vi "Plot Some Cols vs Col N.vi"(1 "Display/hide":bool[](array[boolean]), 2 "Column for abscissa":i32=1 min=0, 3 "Input Array":dbl[][](array[numeric]) format="%.4e") -> (0 "Output Graph":cluster{dbl[], dbl[]}[](graph))   [LabVIEW 2020]
doc: "Plots the 2nd thru Nth columns of the matrix vs the first column in a multiplot graph. Restricted only by LV- or computer memory.\nScott Hannahs, FBNML, Jan 1992"
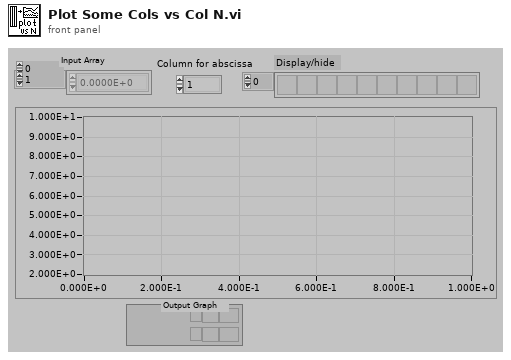
[diagram p1: front panel]
types:
  T1 = cluster{"Input Array":dbl[], "Input Array":dbl[]}
  T2 = cluster{"Input Array":dbl[], "Input Array":dbl[]}[]
  T3 = cluster{"Index Array":dbl[], "Input Array":dbl[]}
  T4 = cluster{"Index Array":dbl[], "Input Array":dbl[]}[]
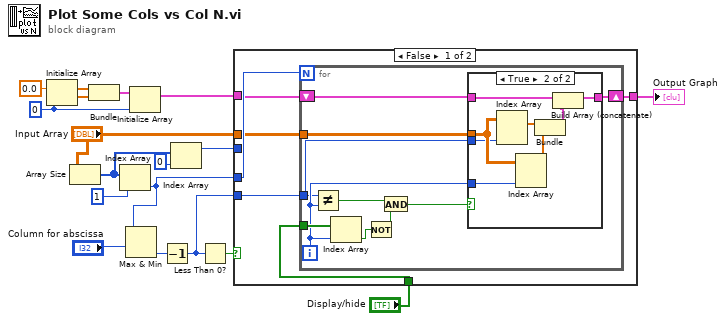
[diagram p0: block diagram]
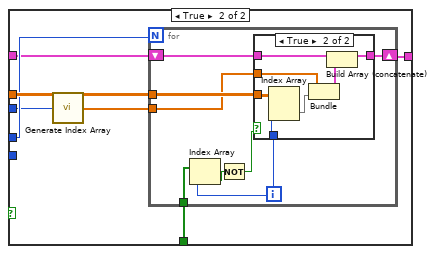
[diagram p3: hidden frame]
diagram:
  w5 = 0
  n1 = Initialize Array(0.0, w5) -> (w8:dbl[])
  n2 = Array Size(array="Input Array") -> (size(s)=w3:i32[])
  n3 = Bundle(w8, w8) -> (w7:cluster{dbl[], dbl[]})  [unwired: 1 in]
  n4 = Index Array(array=w3, index=1) -> (element=w10:i32)
  n5 = Max & Min(x=w10, y="Column for abscissa") -> (min(x,y)=w14:i32)  [unwired: 1 out]
  n6 = Initialize Array(w7, w5) -> (w6:cluster{dbl[], dbl[]}[])
  n7 = Decrement(x=w14) -> (x-1=w16:i32)
  n8 = Index Array(array=w3, index=0) -> (element=w2:i32)
  n9 = Less Than 0?(x=w16) -> (x < 0?=w15:bool)
  n10 = case shown="False" w15 {
    tunnel: w10 -> [w20 w47]
    tunnel: "Display/hide" -> [w22 w48]
    tunnel: [w23 w46] -> w1
    tunnel: w16 -> [w21 _]
    tunnel: "Input Array" -> [w18 w49]
    tunnel: w6 -> [w19 w45]
    tunnel: w2 -> [_ w44]
    frame False {
      n11 = for {
        N: w20 -> [_]
        shift-right: [w32] -> w23
        shift-left: w19 -> [w33]
        tunnel: w22 -> [w29]
        tunnel: w21 -> [w24]
        tunnel: w18 -> [w26]
        i -> [w25]
        n12 = Not Equal?(x=w24, y=w25) -> (x != y?=w30:bool)
        n13 = Index Array(array=w29, index=w25) -> (element=w28:bool)
        n14 = Not(x=w28) -> (.not. x?=w27:bool)
        n15 = And(x=w30, y=w27) -> (x .and. y?=w31:bool)
        n16 = case shown="True" w31 {
          tunnel: [w34 w41] -> w32
          tunnel: w33 -> [w34 w42]
          tunnel: w26 -> [_ w37]
          tunnel: w25 -> [_ w36]
          tunnel: w24 -> [_ w35]
          frame False {
          }
          frame True {
            n17 = Index Array(array=w37, index (col)=w35) -> (element=w39:dbl[])  [unwired: 1 in]
            n18 = Index Array(array=w37, index (col)=w36) -> (element=w38:dbl[])  [unwired: 1 in]
            n19 = Bundle("Input Array"=w39, "Input Array"=w38) -> (w40:T1)  [unwired: 1 in]
            n20 = Build Array (concatenate)(w42, w40) -> (w41:T2)
          }
        }
      }
    }
    frame True {
      n21 = call "Generate Index Array.vi"("Size"=w44) -> ("Index Array"=w43:dbl[])
      n22 = for {
        N: w47 -> [_]
        shift-right: [w56] -> w46
        shift-left: w45 -> [w55]
        tunnel: w48 -> [w54]
        tunnel: w49 -> [w57]
        tunnel: w43 -> [w50]
        i -> [w53]
        n23 = Index Array(array=w54, index=w53) -> (element=w52:bool)
        n24 = Not(x=w52) -> (.not. x?=w51:bool)
        n25 = case shown="True" w51 {
          tunnel: w53 -> [_ w62]
          tunnel: w57 -> [_ w63]
          tunnel: [w58 w64] -> w56
          tunnel: w55 -> [w58 w65]
          tunnel: w50 -> [_ w59]
          frame False {
          }
          frame True {
            n26 = Index Array(array=w63, index (col)=w62) -> (element=w61:dbl[])  [unwired: 1 in]
            n27 = Bundle("Index Array"=w59, "Input Array"=w61) -> (w60:T3)  [unwired: 1 in]
            n28 = Build Array (concatenate)(w65, w60) -> (w64:T4)
          }
        }
      }
    }
  }
  "Output Graph" <- w1
